vi "GOOP4_Sub_Create.vi"(8 "error in (no error)":errorcluster, 9 "Str":string, 10 "i":i32, 11 "reference in":refnum<class "GOOP4_Sub.lvclass">) -> (0 "error out":errorcluster, 3 "reference out":refnum<class "GOOP4_Sub.lvclass">)   [LabVIEW 2016, in "GOOP4_Sub.lvclass"]
uses:
  GOOP4_Sub.lvclass
  C:/Program Files (x86)/National Instruments/LabVIEW 2016/examples/Open_GDS/GDS/GOOP4_CreateObjects_Open_GDS/GOOP4_Base_class/GOOP4_Base.lvclass
  GOOP4_Base_class/GOOP4_Base.lvclass
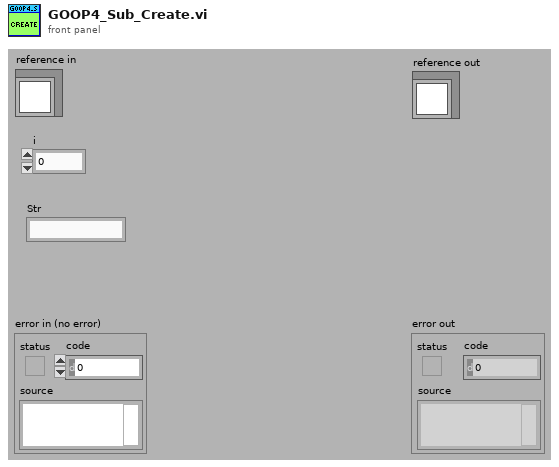
[diagram p1: front panel]
types:
  T1 = typedef "GOOP4_Sub.lvclass/ObjectAttributes.ctl" = cluster{"Str":string}
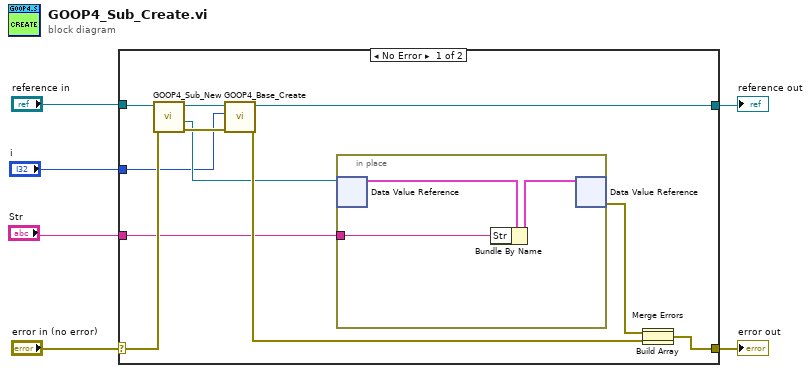
[diagram p0: block diagram]
diagram:
  n1 = case shown="No Error" "error in (no error)" {
    selector: "error in (no error)" -> [w15 w23]
    tunnel: [w13 w23] -> w5
    tunnel: "reference in" -> [w17 w22]
    tunnel: [w12 w22] -> w3
    tunnel: "i" -> [w9 _]
    tunnel: "Str" -> [w8 _]
    frame No Error {
      n2 = call "GOOP4_Sub_New.vi"("error in (no error)"=w15, "reference in"=w17) -> ("error out"=w16:errorcluster, "DVRRefOut"=w10:refnum<data-value>, "reference out"=w18:refnum<class "GOOP4_Sub.lvclass">)  [unwired: 6 in, 1 out]
      n3 = call "GOOP4_Base_Create.vi"("error in (no error)"=w16, "i"=w9, "reference in"=w18) -> ("error out"=w11:errorcluster, "reference out"=w12:refnum<class "GOOP4_Sub.lvclass">)  [unwired: 7 in]
      n4 = in-place {
        in-place-border: w8 -> [w19]
        n5 = in-place-dvr #1(w10) -> (w20:T1)  [unwired: 1 out]
        n6 = Bundle By Name(cluster=w20, "Str"=w19) -> (w21:T1)
        n7 = in-place-dvr #1(w21) -> (w14:errorcluster)  [unwired: 1 out]
      }
      n8 = Build Array(w14, w11) -> (w7:errorcluster[])
      n9 = Merge Errors(w7) -> (w13:errorcluster)
    }
    frame Error {
    }
  }
  "error out" <- w5
  "reference out" <- w3
